vi "USB_CANopenSDODemo.vi"() -> ()   [LabVIEW 2019]
doc: "Read SDO Information.\nThis example is written for a WAGO 750-307 device."
uses:
  <vilib>/nican/nican.llb/xobjhandle.ctl
panel:
  out "ObjHandle out":T1
  in  "Node ID":u8=1
  in  "Baudrate":u32=125000
  in  "Interface":string(combo)="CAN1"
  out "Data":u8[](array[numeric])
  in  "Sub Index":u8 format="%.0x"
  in  "Index":u16=4104 format="%.0x"
  out "Data (ASCII)":string
  out "error out":errorcluster
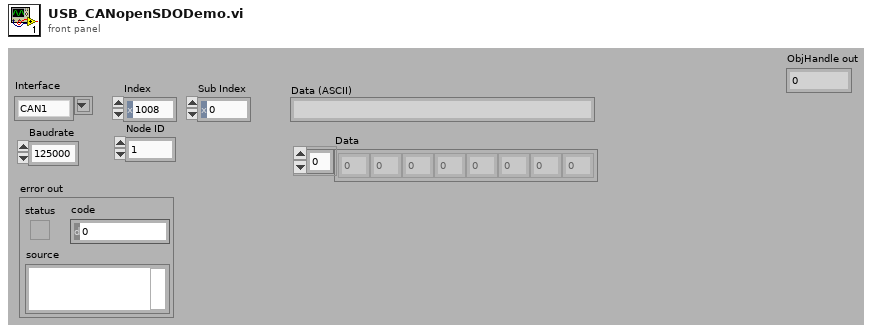
[diagram p1: front panel]
types:
  T1 = typedef "xobjhandle.ctl" = u32
  T2 = enum16{"start remote node", "stop remote node", "reset node", "reset communication", "enter preoperational"}
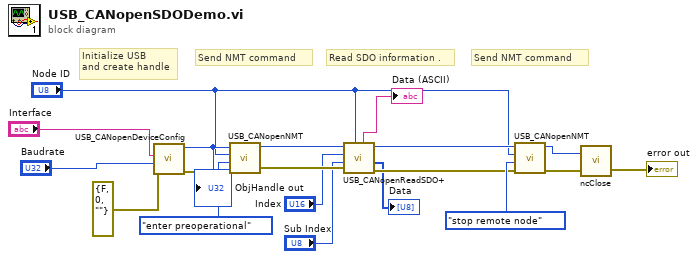
[diagram p0: block diagram]
diagram:
  # "Read SDO information ."
  # "Send NMT command"
  # "Send NMT command"
  # "Initialize USB  \nand create handle"
  n1 = call "USB_CANopenDeviceConfig.vi"("Error in"=errorcluster {"status"=FALSE, "code"=0, "source"=""}, "Baudrate"="Baudrate", "Interface"="Interface") -> ("Error out"=w11:errorcluster, "ObjHandle out"=w7:T1)  [unwired: 7 in]
  "ObjHandle out" <- w7
  n2 = call "USB_CANopenNMT.vi"("error in"=w11, "Mode"=T2."enter preoperational", "Node ID"="Node ID", "ObjHandle in"=w7) -> ("error out"=w17:errorcluster, "ObjHandle out"=w3:T1)  [unwired: 2 in]
  n3 = call "USB_CANopenReadSDO+.vi"("Node ID"="Node ID", "error in"=w17, "Sub Index"="Sub Index", "Index"="Index", "ObjHandle in"=w3) -> ("error out"=w16:errorcluster, "Data"=→"Data":u8[], "ObjHandle out"=w2:T1, "Data (ASCII)"=→"Data (ASCII)":string)  [unwired: 1 in]
  n4 = call "USB_CANopenNMT.vi"("error in"=w16, "Mode"=T2."stop remote node", "Node ID"="Node ID", "ObjHandle in"=w2) -> ("error out"=w6:errorcluster, "ObjHandle out"=w4:T1)  [unwired: 2 in]
  n5 = call <vilib>:"ncClose.vi"("Error in"=w6, "ObjHandle in"=w4) -> ("Error out"=→"error out":errorcluster)  [unwired: 1 in]
